vi "Log Data.vi"(0 "refnum in":refnum<file>, 1 "Temp (C)":dbl, 2 "Heater Status":bool, 3 "Set Point FB":i32 caption="Temp Set Point (C)", 4 "On/Off Set":bool, 5 "Error In":errorcluster) -> (14 "refnum out":refnum<file>, 19 "Error Out":errorcluster)   [LabVIEW 2015]
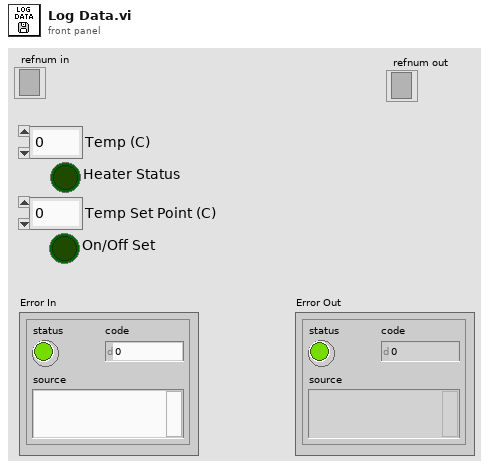
[diagram p1: front panel]
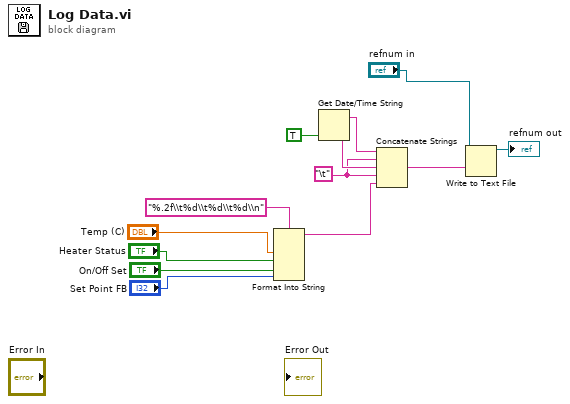
[diagram p0: block diagram]
diagram:
  w9 = "\t"
  n1 = Format Into String(format string="%.2f\\t%d\\t%d\\t%d\\n", "Temp (C)", "Heater Status", "On/Off Set", "Set Point FB") -> (resulting string=w4:string)  [unwired: 2 in, 1 out]
  n2 = Get Date/Time String(want seconds? (F)=TRUE) -> (date string=w12:string, time string=w11:string)  [unwired: 2 in]
  n3 = Concatenate Strings(w12, w9, w11, w9, w4) -> (w10:string)
  n4 = Write to Text File(file (use dialog)="refnum in", text=w10) -> (refnum out=→"refnum out":refnum<file>)  [unwired: 2 in, 2 out]
